vi "init.vi"(8 "error in":errorcluster, 10 "TBM module configuration in":refnum<class "TBM module configuration.lvclass">, 11 "SystemLin Tag Module runtime in":refnum<class "SystemLink File runtime.lvclass">) -> (0 "error out":errorcluster, 1 "data allocations":T1, 2 "execution settings":T4, 3 "SystemLin Tag Module runtime out":refnum<class "SystemLink File runtime.lvclass">)   [LabVIEW 2015, in "SystemLink File runtime.lvclass"]
doc: "Provides an interface for initializing a module at runtime. While this interface performs no operations, a child should provide an override which may open any necessary references or sessions, allocate necessary memory, and perform any final configuration validataion before providing the full configuration <b>execution data</b> to the calling process."
uses:
  SystemLink File runtime.lvclass
  <vilib>/NI/Tag Bus Module Framework/module configuration/TBM module configuration.lvclass
  <vilib>/NI/Tag Bus Module Framework/runtime/execution settings.ctl
  <vilib>/NI/Tag Bus Module Framework/channel/data tables.ctl
  <vilib>/NI/Tag Bus/dictionary/data dictionary.lvclass
  <vilib>/NI/Tag Bus/dictionary table pair.ctl
  <vilib>/NI/Tag Bus/table/data table.ctl
  configuration/SystemLink File configuration.lvclass
  configuration/SystemLink File configuration.lvclass/SystemLink File configuration.ctl
  <vilib>/NI/Tag Bus/tag/tag descriptor.lvclass/tag descriptor.ctl
  SystemLink File runtime.lvclass/SystemLink File runtime.ctl
  configuration/Read Connection Configuration.vi
  <vilib>/NI/Tag Bus/tag/read tag name.vi
  <vilib>/NI/Tag Bus/tag/read data type.vi
  <vilib>/NI/Tag Bus/dictionary/locate tag.vi
  <vilib>/NI/Tag Bus Module Framework/channel/TBM channel.lvclass
  <vilib>/NI/Tag Bus Module Framework/runtime/TBM module execution interface.lvclass
  <vilib>/NI/Tag Bus/tag bus.lvlib
  <vilib>/NI/Tag Bus/table/data table.lvlib
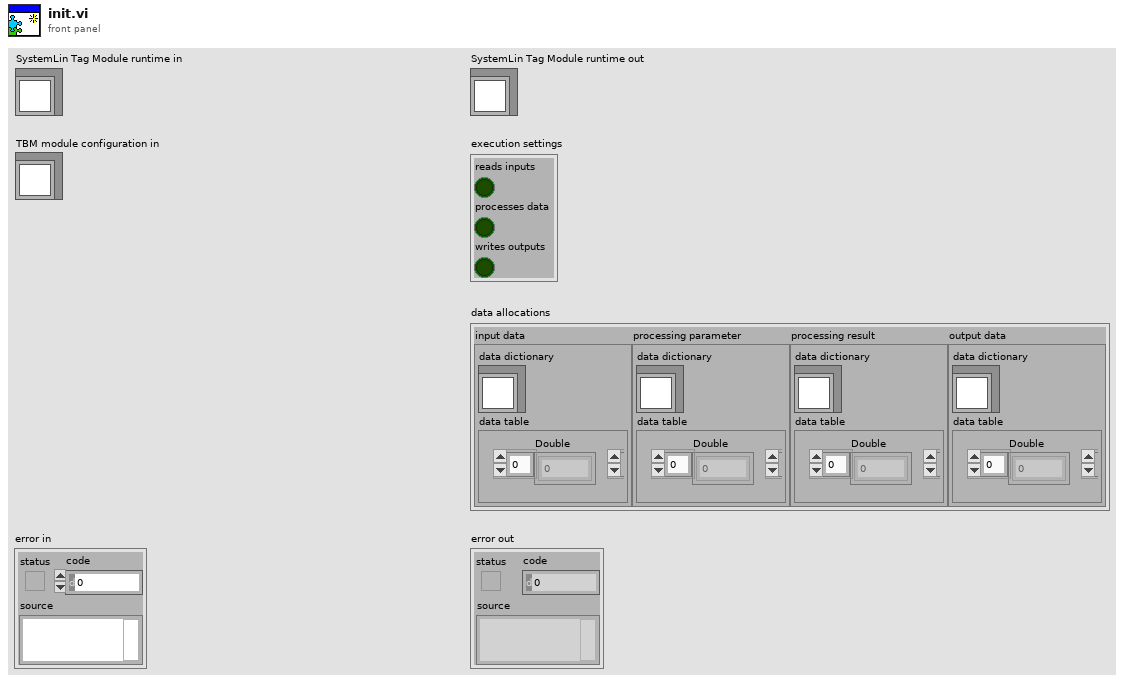
[diagram p1: front panel]
types:
  T1 = typedef "TBM channel.lvclass/data tables.ctl" = cluster{"input data":T2, "processing parameter":T2, "processing result":T2, "output data":T2}
  T2 = typedef "tag bus.lvlib/dictionary table pair.ctl" = cluster{"data dictionary":refnum<class "data dictionary.lvclass">, "data table":T3}
  T3 = typedef "tag bus.lvlib/data table.lvlib/data table.ctl" = cluster{"Double":dbl[], "Single":sgl[], "I64":i64[], "I32":i32[], "I16":i16[], "I8":i8[], "U64":u64[], "U32":u32[], "U16":u16[], "U8":u8[], "Boolean":bool[], "String":string[], "Array of Double":cluster{"DBL Array":dbl[]}[], "Array of Single":cluster{"SGL Array":sgl[]}[], "Array of I64":cluster{"I64 Array":i64[]}[], "Array of I32":cluster{"I32 Array":i32[]}[], "Array of I16":cluster{"I16 Array":i16[]}[], "Array of I8":cluster{"I8 Array":i8[]}[], "Array of U64":cluster{"U64 Array":u64[]}[], "Array of U32":cluster{"U32 Array":u32[]}[], "Array of U16":cluster{"U16 Array":u16[]}[], "Array of U8":cluster{"U8 Array":u8[]}[], "Array of Boolean":cluster{"Boolean Array":bool[]}[], "Array of String":cluster{"String Array":string[]}[]}
  T4 = typedef "TBM module execution interface.lvclass/execution settings.ctl" = cluster{"reads inputs":bool, "processes data":bool, "writes outputs":bool}
  T5 = typedef "SystemLink File configuration.lvclass/Connection Configuration.ctl" = cluster{"Connection Type":T6, "AMQP":cluster{"Configuration ID":string}, "HTTP":cluster{"Verify Server?":bool, "Server URL":string, "CA Certificate File":string, "User Info":cluster{"Username":string, "Password":string}, "API Key":string}}
  T6 = typedef "SystemLink File configuration.lvclass/Connection Type.ctl" = enum16{"AMQP", "HTTP", "API Key (SystemLink Cloud)"}
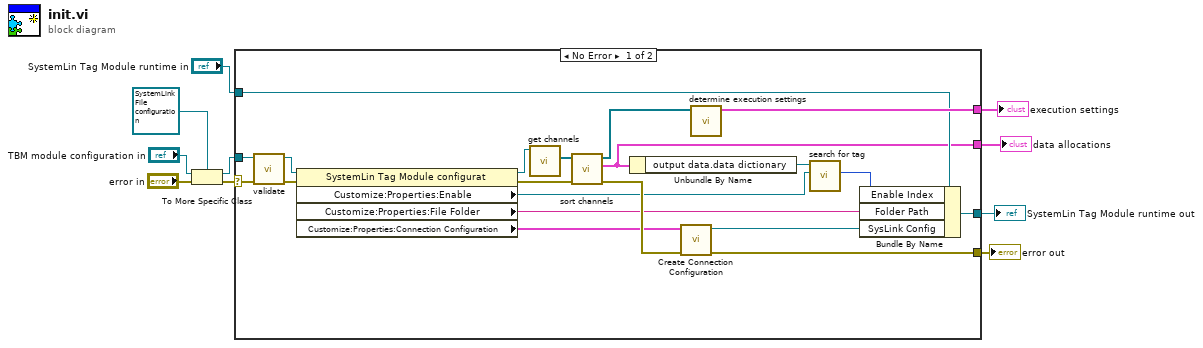
[diagram p0: block diagram]
diagram:
  n1 = To More Specific Class(target class=refnum<class "SystemLink File configuration.lvclass"> refnum ("Synchronous module configuration"), reference="TBM module configuration in", error in="error in") -> (specific class reference=w9:refnum<class "SystemLink File configuration.lvclass">, error out=w10:errorcluster)
  n2 = case shown="No Error" w10 {
    selector: w10 -> [w29 w31]
    tunnel: w9 -> [w28 _]
    tunnel: "SystemLin Tag Module runtime in" -> [w25 w32]
    tunnel: [w24 w32] -> w4
    tunnel: [w13 w31] -> w3
    tunnel: [w22 _] -> w1
    tunnel: [w30 _] -> w2
    frame No Error {
      n3 = call-dynamic "validate.vi"("error in"=w29, "SystemLin Tag Module configuration in"=w28) -> ("error out"=w18:errorcluster, "SystemLin Tag Module configuration out"=w21:refnum<class "SystemLink File configuration.lvclass">)  [unwired: 8 in]
      n4 = property class="SystemLin Tag Module configurat"(reference=w21, error in=w18) -> (reference out=w20:refnum<class "SystemLink File configuration.lvclass">, error out=w17:errorcluster, "Customize:Properties:Enable"=w16:refnum<class "TBM channel.lvclass">, "Customize:Properties:File Folder"=w14:string, "Customize:Properties:Connection Configuration"=w12:T5)
      n5 = call-dynamic "get channels.vi"("SystemLin Tag Module configuration in"=w20) -> ("channels"=w27:refnum<class "TBM channel.lvclass">[])  [unwired: 9 in, 1 out]
      n6 = call <vilib>:"sort channels.vi"("error in"=w17, "channels in"=w27) -> ("error out"=w23:errorcluster, "data allocations"=w22:T1, "channels out"=w26:refnum<class "TBM channel.lvclass">[])  [unwired: 7 in]
      n7 = Unbundle By Name(w22) -> ("output data.data dictionary"=w19:refnum<class "data dictionary.lvclass">)
      n8 = call "Create Connection Configuration.vi"("error in (no error)"=w23, "Connection Configuration"=w12) -> ("error out"=w13:errorcluster, "SystemLink Configuration"=w11:refnum<class "NI Skyline Configuration.lvclass">)  [unwired: 8 in]
      n9 = call <vilib>:"determine execution settings.vi"("channels"=w26) -> ("execution settings"=w30:T4)  [unwired: 10 in]
      n10 = call <vilib>:"search for tag.vi"("system tag"=w16, "data dictionary in"=w19) -> ("index"=w15:i32)  [unwired: 7 in, 2 out]
      n11 = Bundle By Name(cluster=w25, "Enable Index"=w15, "Folder Path"=w14, "SysLink Config"=w11) -> (w24:refnum<class "SystemLink File runtime.lvclass">)
    }
    frame Error {
    }
  }
  "error out" <- w3
  "SystemLin Tag Module runtime out" <- w4
  "execution settings" <- w2
  "data allocations" <- w1
